vi "SVL AC & DC Level (1 Ch SGL WDT).vi"(9 "window":u16(ring)=8 items=["None ", "Hanning", "Hamming", "Blackman-Harris", "Exact Blackman", "Blackman", "Flat Top", "4 Term B-Harris ", "7 Term B-Harris", "Low Sidelobe"], 11 "scaled signal [EU]":waveform(sgl)={"t0"=timestamp(0 s since 1904-01-01), "dt"=0.0, "Y"=[]}) -> (1 "DC level [EU]":dbl=nan format="%0.2f", 2 "AC level [EU rms]":dbl=nan format="%.8f", 3 "AC signal [EU]":waveform(sgl))   [LabVIEW 2017]
doc: "Computes the AC level and DC level of a signal. Wire data to the <B>scaled signal [EU]</B> input to determine the polymorphic instance to use or manually select the instance."
uses:
  <vilib>/Analysis/4window.llb/windowTd.ctl
  <vilib>/Analysis/baseanly.llb/Mean (DBL).vi
  <vilib>/Analysis/0measdsp.llb/Scaled Time Domain Window (DBL).vi
  <vilib>/Analysis/NI_AALBase.lvlib
  <vilib>/Analysis/NI_AALPro.lvlib
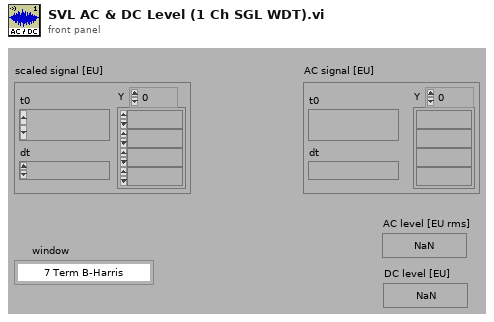
[diagram p1: front panel]
types:
  T1 = typedef "NI_AALPro.lvlib/windowTd.ctl" = u32
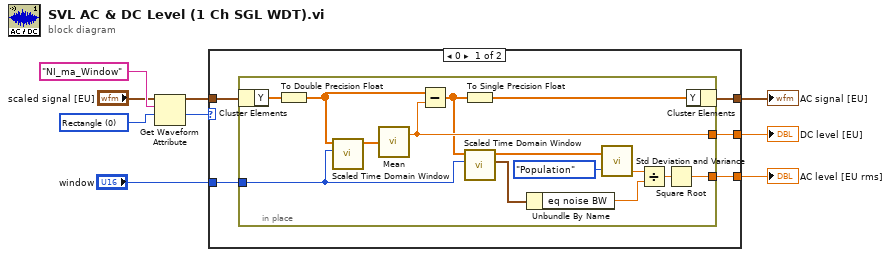
[diagram p0: block diagram]
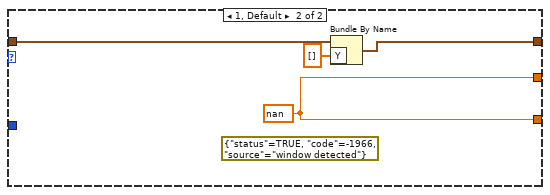
[diagram p2: hidden frame]
diagram:
  w4 = T1 0 items=["Rectangle"=0, "Hanning"=1, "Hamming"=2, "Blackman-Harris"=3, "Exact Blackman"=4, "Blackman"=5, "Flat Top"=6, "4 Term B-Harris "=7, "7 Term B-Harris"=8, "Low Sidelobe"=9, "Blackman Nuttall"=11, "Triangle"=30, "Bartlett-Hanning"=31, "Bohman"=32, "Parzen"=33, "Welch"=34, "Kaiser"=60, "Dolph-Chebyshev"=61, "Gaussian"=62] ("window")
  n1 = Get Waveform Attribute(5:w4, 6:"NI_ma_Window" ("name"), 7:"scaled signal [EU]") -> (1:w1:T1, 3:w2:waveform(sgl))  [unwired: 1 in, 2 out]
  n2 = case shown="0" w1 {
    tunnel: [w13 w32] -> w9
    tunnel: [w12 w32] -> w6
    tunnel: "window" -> [w14 _]
    tunnel: [w11 w30] -> w7
    tunnel: w2 -> [w10 w31]
    frame 0 {
      n3 = in-place {
        in-place-border: [w22] -> w12
        in-place-border: w14 -> [w17]
        in-place-border: [w23] -> w13
        n4 = in-place-cluster #1(w10) -> ("Y"=w28:sgl[])
        n5 = To Double Precision Float(number=w28) -> (double precision float=w15:dbl[])
        n6 = call-poly <vilib>:"Scaled Time Domain Window.vi"("window"=w17, "X"=w15) -> ("Windowed X"=w21:dbl[])  [unwired: 7 in, 2 out]
        n7 = call-poly <vilib>:"Mean.vi"("X"=w21) -> ("mean"=w22:dbl)  [unwired: 1 out]
        n8 = Subtract(x=w15, y=w22) -> (x-y=w19:dbl[])
        n9 = To Single Precision Float(number=w19) -> (single precision float=w16:sgl[])
        n10 = call-poly <vilib>:"Scaled Time Domain Window.vi"("window"=w17, "X"=w19) -> ("window properties"=w18:cluster{"eq noise BW":dbl, "coherent gain":dbl}, "Windowed X"=w20:dbl[])  [unwired: 7 in, 1 out]
        n11 = Unbundle By Name(w18) -> ("eq noise BW"=w24:dbl)
        n12 = call <vilib>:"Std Deviation and Variance.vi"("X"=w20, "Weighting (Sample)"=enum16{"Sample", "Population"}."Population") -> ("variance"=w27:dbl)  [unwired: 2 out]
        n13 = Divide(x=w27, y=w24) -> (x/y=w25:dbl)
        n14 = Square Root(x=w25) -> (sqrt(x)=w23:dbl)
        n15 = in-place-cluster #1("Y"=w16) -> (w11:waveform(sgl))
      }
    }
    frame 1, Default {
      w32 = nan ("mean")
      (unwired) errorcluster {"status"=TRUE, "code"=-1966, "source"="window detected"} ("error in 2 (no error)")
      n16 = Bundle By Name(cluster=w31, "Y"=dbl[] []) -> (w30:waveform(sgl))
    }
  }
  "AC level [EU rms]" <- w9
  "DC level [EU]" <- w6
  "AC signal [EU]" <- w7
